vi "Dialog Sandbox.vi"() -> ()   [LabVIEW 2021, in "Settings.lvlib"]
uses:
  Acquisition/IO Device.ctl
  Acquisition/Sensor Type.ctl
  Settings.lvlib
  Acquisition/Acquisition.lvlib
panel:
  in  "Calibration Settings":T1(array[cluster])
  in  "Channel Settings":T4(array[cluster])
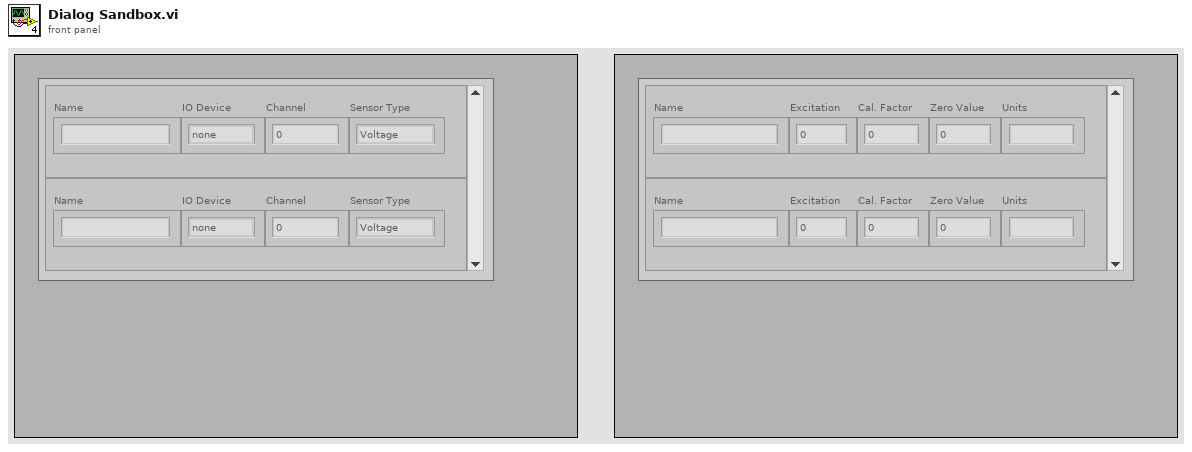
[diagram p1: front panel]
types:
  T1 = cluster{"Name":string, "Calibration Information":cluster{"Excitation":dbl, "Cal. Factor":dbl, "Zero Value":dbl, "Units":string}}[]
  T2 = typedef "Acquisition.lvlib/IO Device.ctl" = enum16{"none", "9219", "9401"}
  T3 = typedef "Acquisition.lvlib/Sensor Type.ctl" = enum16{"Voltage", "Load", "Pressure", "Encoder"}
  T4 = cluster{"Name":string, "Terminal Information":cluster{"IO Device":T2, "Channel":i32, "Sensor Type":T3}}[]
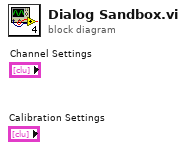
[diagram p0: block diagram]
diagram:
